vi "transientTriggeredEx.vi"() -> ()   [LabVIEW 2017]
uses:
  <instrlib>/BK Precision 85XX Series/BK Precision 85XX Series.lvlib
panel:
  in  "Mode of Operation (0:CC)":u16(ring)=3 items=["CC", "CV", "CW", "CR"]
  out "error out":errorcluster
  out "Terminal Input Power (W)":dbl(graph)
  out "Terminal Input Current (A)":dbl(graph)
  out "Terminal Input Voltage (V)":dbl(graph)
  in  "Communication Address (0)":u8 max=254 format="%x"
  in  "loop time (ms)":u32=500
  in  "stop":bool
  in  "Enable Input Terminals (F: Off)":bool=TRUE
  out "Trigger Source (0=immediate, 1=external, 2=bus)":u8
  in  "Transient Operation (0:Continuous)":u8(ring) items=["Continuous", "Pulse", "Toggled"]
  in  "Level B Timing (0.5)":dbl=0.5 min=0.5 max=6000.0 step=0.5 format="%#_5g"
  in  "Level B Value (0)":dbl min=0.0 max=6000.0
  in  "Level A Timing (0.5)":dbl=0.5 min=0.5 max=6000.0 step=0.5 format="%#_5g"
  in  "Level A Value (0)":dbl min=0.0 max=6000.0
  out "Serial Number":string
  out "Product Model":string
  out "Firmware Version":string
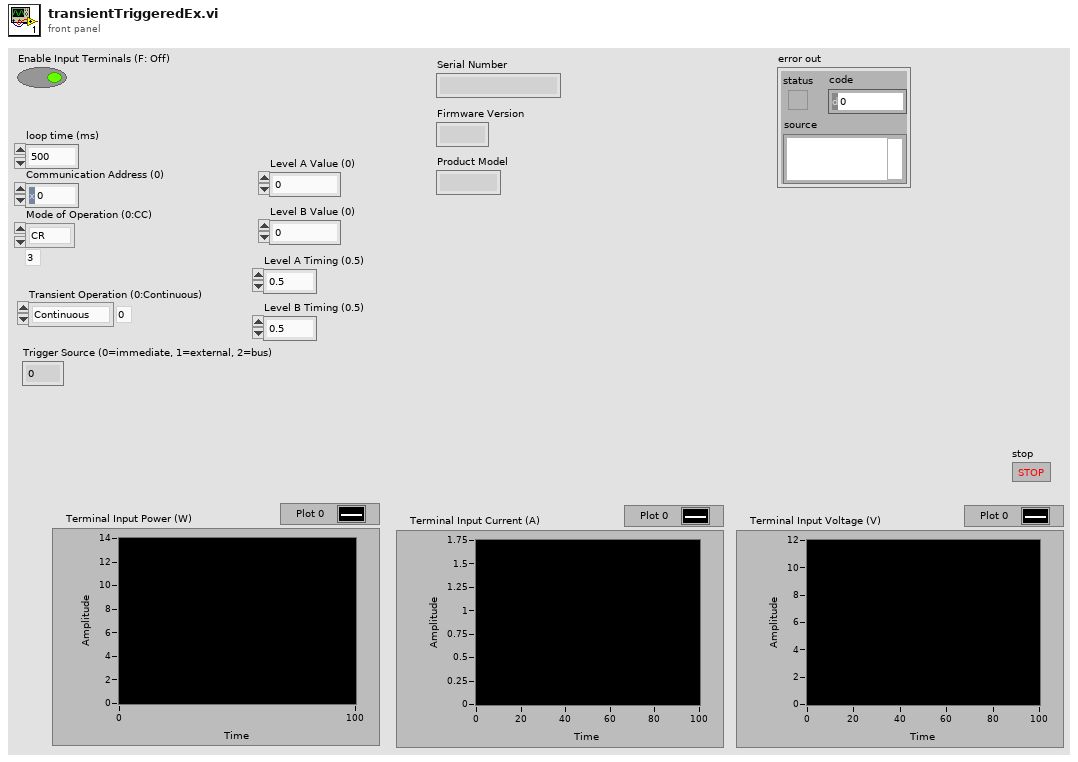
[diagram p1: front panel]
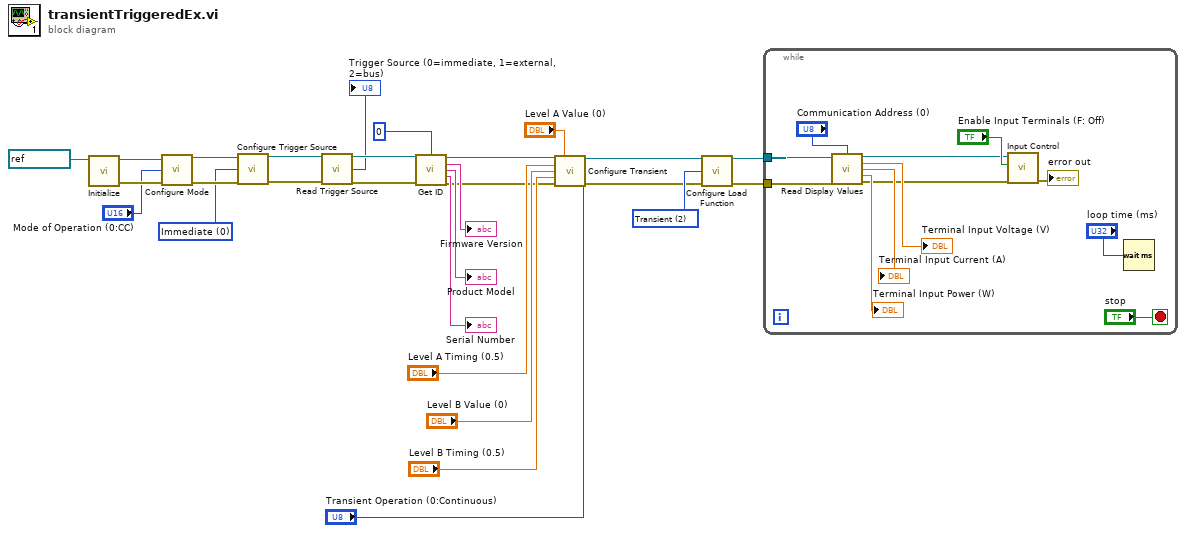
[diagram p0: block diagram]
diagram:
  w5 = u16 2 items=["Fixed", "Short", "Transient", "List", "Battery"] ("Function (0:FIXED)")
  w13 = u8 0 items=["Immediate", "External", "Bus"] ("Trigger Source (0:Immediate)")
  n1 = call <instrlib>:"Initialize.vi"("VISA resource name"=refnum<visa-resource-name> "COM4") -> ("error out"=w17:errorcluster, "VISA resource name out"=w18:refnum<visa-resource-name>)  [unwired: 9 in]
  n2 = call <instrlib>:"Configure Mode.vi"("VISA resource name"=w18, "Mode of Operation (0:CC)"="Mode of Operation (0:CC)", "error in (no error)"=w17) -> ("VISA resource name out"=w14:refnum<visa-resource-name>, "error out"=w15:errorcluster)  [unwired: 11 in]
  n3 = call <instrlib>:"Configure Trigger Source.vi"("VISA resource name"=w14, "Trigger Source (0:Immediate)"=w13, "error in (no error)"=w15) -> ("VISA resource name out"=w12:refnum<visa-resource-name>, "error out"=w9:errorcluster)  [unwired: 11 in]
  n4 = call <instrlib>:"Read Trigger Source.vi"("VISA resource name"=w12, "error in (no error)"=w9) -> ("VISA resource name out"=w11:refnum<visa-resource-name>, "Trigger Source"=→"Trigger Source (0=immediate, 1=external, 2=bus)":u8, "error out"=w10:errorcluster)  [unwired: 11 in]
  n5 = call <instrlib>:"Get ID.vi"("VISA resource name"=w11, "Communication Address (0)"=u8 0, "error in (no error)"=w10) -> ("VISA resource name out"=w7:refnum<visa-resource-name>, "Firmware Version"=→"Firmware Version":string, "Product Model"=→"Product Model":string, "Serial Number"=→"Serial Number":string, "error out"=w6:errorcluster)  [unwired: 8 in]
  n6 = call <instrlib>:"Configure Transient.vi"("VISA resource name"=w7, "Level A Value (0)"="Level A Value (0)", "Level A Timing (0.5)"="Level A Timing (0.5)", "Level B Value (0)"="Level B Value (0)", "Level B Timing (0.5)"="Level B Timing (0.5)", "error in (no error)"=w6, "Transient Operation (0:Continuous)"="Transient Operation (0:Continuous)") -> ("VISA resource name out"=w2:refnum<visa-resource-name>, "error out"=w1:errorcluster)  [unwired: 7 in]
  n7 = call <instrlib>:"Configure Load Function.vi"("VISA resource name"=w2, "Function (0:FIXED)"=w5, "error in (no error)"=w1) -> ("VISA resource name out"=w4:refnum<visa-resource-name>, "error out"=w3:errorcluster)  [unwired: 11 in]
  n8 = while {
    tunnel: w4 -> [w37]
    tunnel: w3 -> [w31]
    stop <- "stop" stop-if-true
    n9 = call <instrlib>:"Read Display Values.vi"("VISA resource name"=w37, "Communication Address (0)"="Communication Address (0)", "error in (no error)"=w31) -> ("VISA resource name out"=w36:refnum<visa-resource-name>, "Terminal Input Voltage (V)"=→"Terminal Input Voltage (V)":dbl, "Terminal Input Current (A)"=→"Terminal Input Current (A)":dbl, "Terminal Input Power (W)"=→"Terminal Input Power (W)":dbl, "error out"=w30:errorcluster)  [unwired: 8 in]
    n10 = call <instrlib>:"Input Control.vi"("error in (no error)"=w30, "Enable Input Terminals (F: Off)"="Enable Input Terminals (F: Off)", "VISA resource name"=w36) -> ("error out"=→"error out":errorcluster)  [unwired: 7 in, 1 out]
    n11 = Wait (ms)(milliseconds to wait="loop time (ms)") -> ()  [unwired: 1 out]
  }
